vi "PCO_SC2_Hardware_Struct.vi"() -> (0 "PCO_SC2_HW_Desc":T1, 1 "PCO_SC2_HW_Desc_Raw":T2, 2 "Length":u16, 3 "Raw_Length":u16)   [LabVIEW 2020, in "SDK.lvlib" / "Structures.lvlib"]
doc: "Use this template to build a VI to use as a subVI."
uses:
  Structures.lvlib
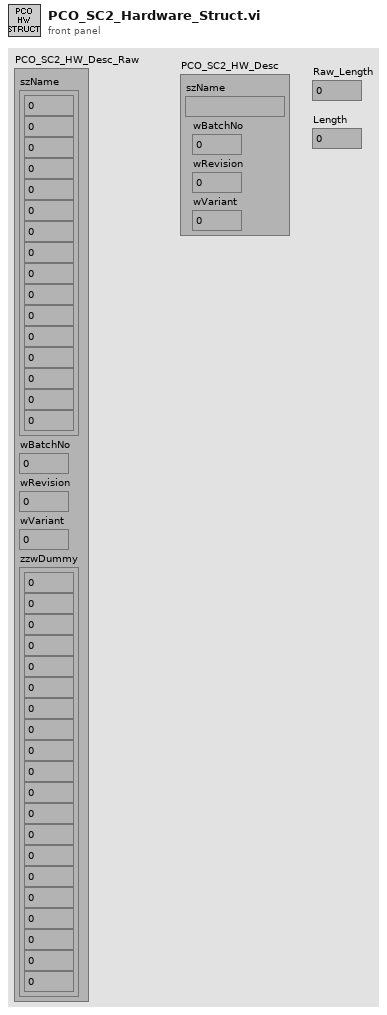
[diagram p1: front panel]
types:
  T1 = cluster{"szName":string, "wBatchNo":u16, "wRevision":u16, "wVariant":u16}
  T2 = cluster{"szName":cluster{u8, u8, u8, u8, u8, u8, u8, u8, u8, u8, u8, u8, u8, u8, u8, u8}, "wBatchNo":u16, "wRevision":u16, "wVariant":u16, "zzwDummy":cluster{u16, u16, u16, u16, u16, u16, u16, u16, u16, u16, u16, u16, u16, u16, u16, u16, u16, u16, u16, u16}}
  T3 = cluster{u16, u16, u16, u16, u16, u16, u16, u16, u16, u16, u16, u16, u16, u16, u16, u16, u16, u16, u16, u16}
  T4 = cluster{u8, u8, u8, u8, u8, u8, u8, u8, u8, u8, u8, u8, u8, u8, u8, u8}
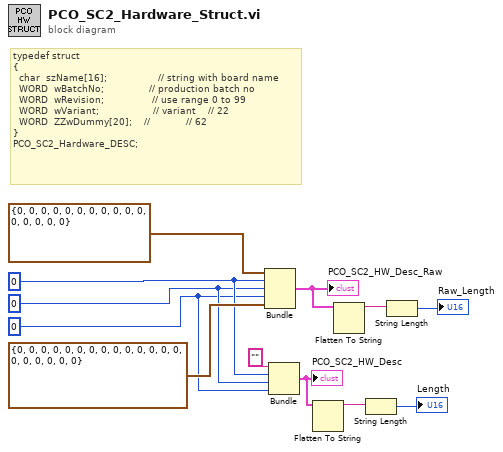
[diagram p0: block diagram]
diagram:
  w7 = u16 0 ("wVariant")
  w8 = u16 0 ("wRevision")
  w9 = u16 0 ("wBatchNo")
  # "typedef struct\n{\n  char  szName[16];                 // string with board name\n  WORD  wBatchNo;               // production batch no\n  WORD  wRevision;                // use range 0 to 99\n  WORD  wVariant;                  // variant    // 22\n  WORD  ZZwDummy[20];    //            // 62\n}\nPCO_SC2_Hardware_DESC;"
  n1 = Bundle("szName"=T4 {0, 0, 0, 0, 0, 0, 0, 0, 0, 0, 0, 0, 0, 0, 0, 0}, "wBatchNo"=w9, "wRevision"=w8, "wVariant"=w7, "zzwDummy"=T3 {0, 0, 0, 0, 0, 0, 0, 0, 0, 0, 0, 0, 0, 0, 0, 0, 0, 0, 0, 0}) -> (w1:T2)  [unwired: 1 in]
  "PCO_SC2_HW_Desc_Raw" <- w1
  n2 = Bundle("szName"="", "wBatchNo"=w9, "wRevision"=w8, "wVariant"=w7) -> (w4:T1)  [unwired: 1 in]
  "PCO_SC2_HW_Desc" <- w4
  n3 = Flatten To String(anything=w4) -> (data string=w6:string)  [unwired: 3 in, 2 out]
  n4 = Flatten To String(anything=w1) -> (data string=w3:string)  [unwired: 3 in, 2 out]
  n5 = String Length(string=w6) -> (length=→"Length":i32)
  n6 = String Length(string=w3) -> (length=→"Raw_Length":i32)
